vi "User Event.vi"(0 "User data":bool, 11 "Error in":errorcluster, 13 "Operation":T1) -> (4 "user event":refnum<user-event>, 15 "Error out":errorcluster)   [LabVIEW 2020, in "Simple calculator.lvlib"]
doc: "This Vi is used a user event LV2 for generating and creating user events."
uses:
  Simple calculator.lvlib
  Typedefs/User event operations.ctl
panel:
  # "USER EVENT LV2"
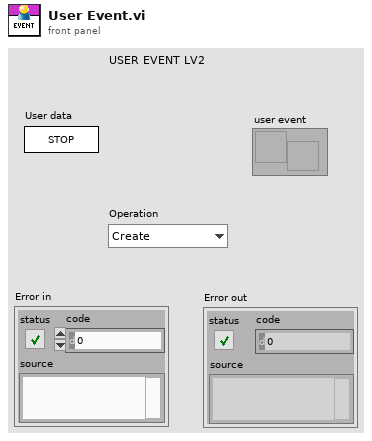
[diagram p1: front panel]
types:
  T1 = typedef "User event operations.ctl" = enum16{"Create", "Get Ref", "Generate ", "Destroy"}
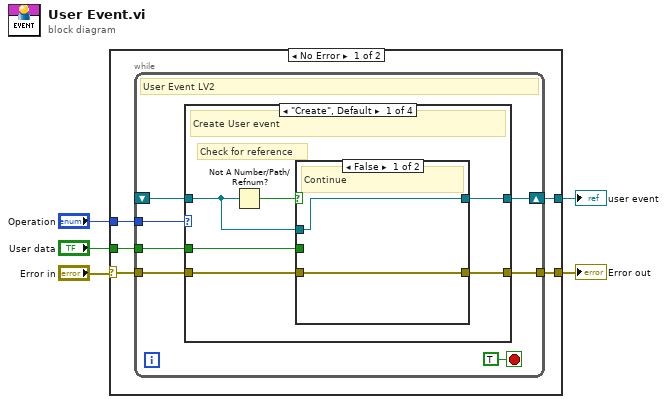
[diagram p0: block diagram]
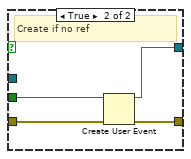
[diagram p2: hidden frame]
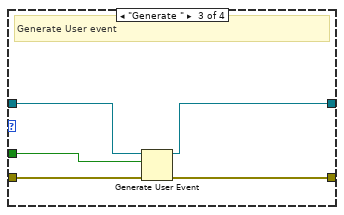
[diagram p4: hidden frame]
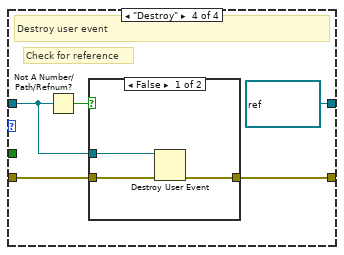
[diagram p5: hidden frame]
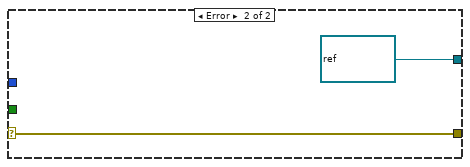
[diagram p7: hidden frame]
diagram:
  n1 = case shown="No Error" "Error in" {
    selector: "Error in" -> [w10 w47]
    tunnel: "Operation" -> [w9 _]
    tunnel: [w8 w47] -> w3
    tunnel: "User data" -> [w7 _]
    tunnel: [w6 refnum<user-event> refnum ("user event")] -> w1
    frame No Error {
      n2 = while {
        tunnel: w10 -> [w15]
        tunnel: w9 -> [w16]
        tunnel: [w14] -> w8
        shift-right: [w13] -> w6
        shift-left: _ -> [w12]
        tunnel: w7 -> [w11]
        stop <- TRUE stop-if-true
        # "User Event LV2"
        n3 = case shown="\"Create\", Default" w16 {
          tunnel: [w22 w31 w35 w40] -> w14
          tunnel: w15 -> [w23 w31 w36 w41]
          tunnel: [w21 w30 w34 refnum<user-event> refnum ("user event")] -> w13
          tunnel: w12 -> [w19 w30 w33 w37]
          tunnel: w11 -> [w18 _ w32 _]
          frame "Create", Default {
            # "Check for reference"
            # "Create User event"
            n4 = Not A Number/Path/Refnum?(number/path/refnum=w19) -> (NaN/Path/Refnum?=w20:bool)
            n5 = case shown="False" w20 {
              tunnel: w23 -> [w25 w29]
              tunnel: [w25 w28] -> w22
              tunnel: [w24 w27] -> w21
              tunnel: w19 -> [w24 _]
              tunnel: w18 -> [_ w26]
              frame False {
                # "Continue"
              }
              frame True {
                # "Create if no ref"
                n6 = Create User Event(user event datatype=w26, error in=w29) -> (user event=w27:refnum<user-event>, error out=w28:errorcluster)
              }
            }
          }
          frame "Get Ref" {
            # "Get User event reference"
          }
          frame "Generate " {
            # "Generate User event"
            n7 = Generate User Event(user event=w33, event data cluster=w32, error in=w36) -> (user event out=w34:refnum<user-event>, error out=w35:errorcluster)  [unwired: 1 in]
          }
          frame "Destroy" {
            # "Check for reference"
            # "Destroy user event"
            n8 = Not A Number/Path/Refnum?(number/path/refnum=w37) -> (NaN/Path/Refnum?=w38:bool)
            n9 = case shown="False" w38 {
              tunnel: w41 -> [w44 w45]
              tunnel: [w43 w45] -> w40
              tunnel: w37 -> [w42 _]
              frame False {
                n10 = Destroy User Event(user event=w42, error in=w44) -> (error out=w43:errorcluster)
              }
              frame True {
              }
            }
          }
        }
      }
    }
    frame Error {
    }
  }
  "Error out" <- w3
  "user event" <- w1
